vi "Find APU Channels.vi"(7 "Custom Device Ref":T1 format="%.0x", 8 "error in (no error)":errorcluster, 9 "Channel Descriptors in":T2, 11 "APU ref":T1 format="%.0x") -> (0 "error out":errorcluster, 1 "Channel Descriptors out":T2)   [LabVIEW 2011, in "Engine Sim System Explorer.lvlib"]
uses:
  Engine Sim System Explorer.lvlib
  <vilib>/NI Veristand/Custom Device API/Custom Device Item Ref.ctl
  Shared/Channel Descriptors.ctl
  Shared/FPGA Write Descriptor.ctl
  Shared/InputChannelTypes.ctl
  <vilib>/rvi/DataTransferAndStorage/Container/Common/niFpgaDataTypeControl.ctl
  Shared/FPGA Read Descriptor.ctl
  Shared/OutputChannelTypes.ctl
  Shared/Status Chan Descriptor.ctl
  <vilib>/NI Veristand/Custom Device Tools/Custom Device Utility Library/NI VeriStand - Search for Item by Name.vi
  <vilib>/NI Veristand/Custom Device Tools/Custom Device Utility Library/Custom Device Utility Library.lvlib
  Engine Simulation Shared.lvlib
  <vilib>/NI Veristand/Custom Device API/Custom Device API.lvlib
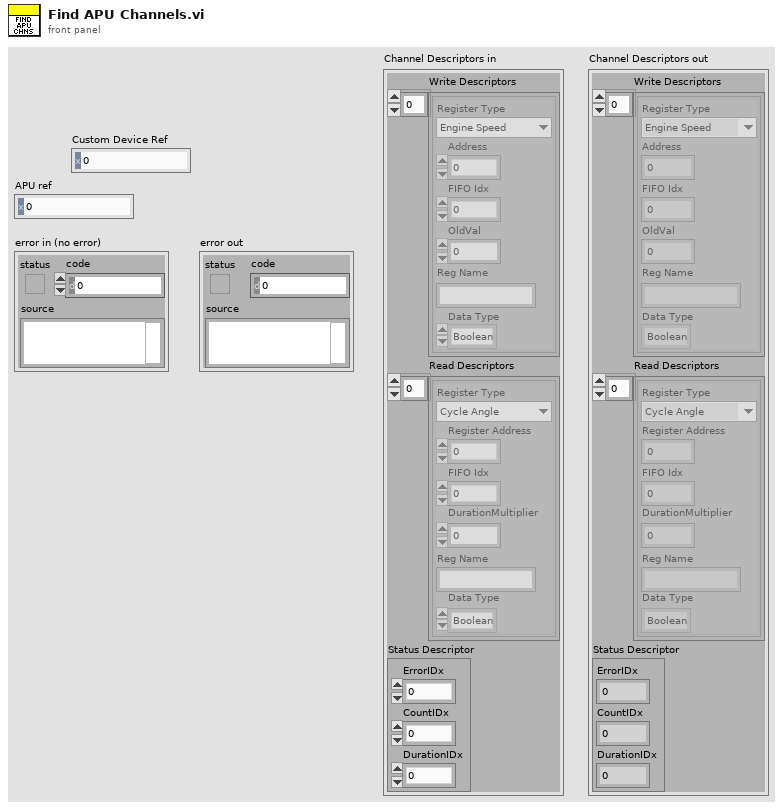
[diagram p1: front panel]
types:
  T1 = typedef "Custom Device API.lvlib/Custom Device Item Ref.ctl" = u64
  T2 = typedef "Engine Simulation Shared.lvlib/Channel Descriptors.ctl" = cluster{"Write Descriptors":T3[], "Read Descriptors":T6[], "Status Descriptor":T8}
  T3 = typedef "Engine Simulation Shared.lvlib/FPGA Write Descriptor.ctl" = cluster{"Register Type":T4, "Address":u32, "FIFO Idx":i32, "OldVal":dbl, "Reg Name":string, "Data Type":T5}
  T4 = typedef "Engine Simulation Shared.lvlib/InputChannelTypes.ctl" = enum16{"Engine Speed", "Offset"}
  T5 = typedef "niFpgaDataTypeControl.ctl" = enum32{"Boolean", "I8", "I16", "I32", "I64", "U8", "U16", "U32", "U64", "FXP", "CustomControl"}
  T6 = typedef "Engine Simulation Shared.lvlib/FPGA Read Descriptor.ctl" = cluster{"Register Type":T7, "Register Address":u32, "FIFO Idx":i32, "DurationMultiplier":dbl, "Reg Name":string, "Data Type":T5}
  T7 = typedef "Engine Simulation Shared.lvlib/OutputChannelTypes.ctl" = enum16{"Cycle Angle", "Crank Angle", "Time Duration", "Angle Duration", "Start Angle", "End Angle"}
  T8 = typedef "Engine Simulation Shared.lvlib/Status Chan Descriptor.ctl" = cluster{"ErrorIDx":i32, "CountIDx":i32, "DurationIDx":i32}
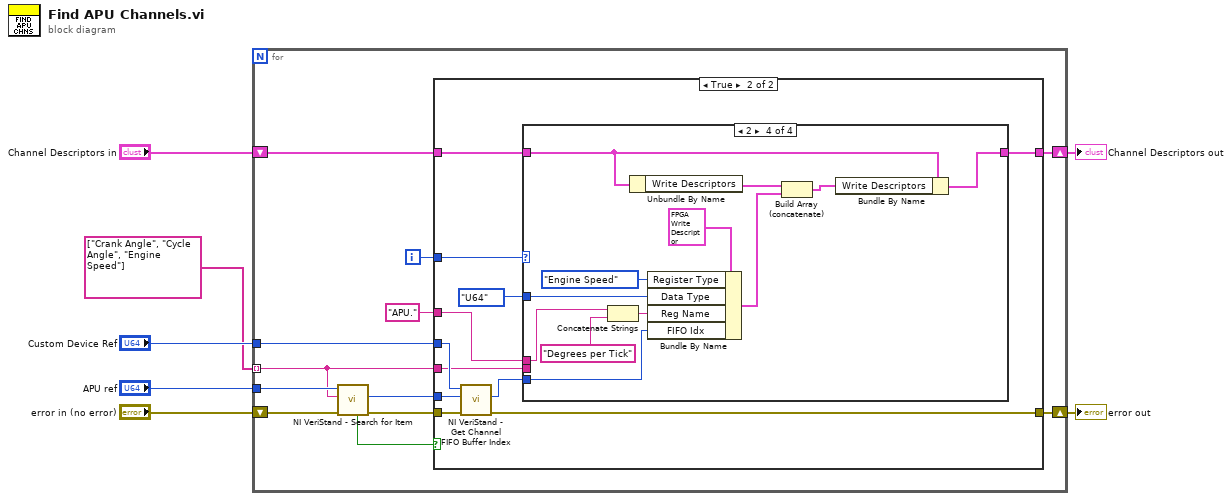
[diagram p0: block diagram]
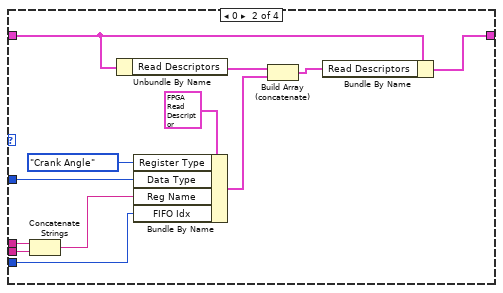
[diagram p4: hidden frame]
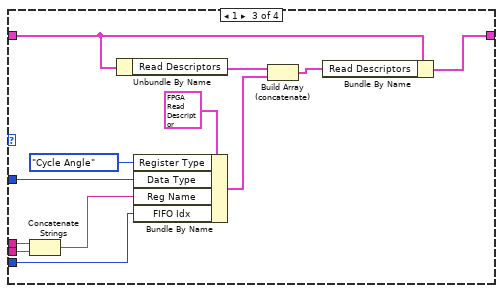
[diagram p5: hidden frame]
diagram:
  n1 = for {
    tunnel: "APU ref" -> [w19]
    tunnel: "Custom Device Ref" -> [w12]
    shift-right: [w9] -> w1
    shift-left: "error in (no error)" -> [w18]
    shift-right: [w11] -> w3
    shift-left: "Channel Descriptors in" -> [w13]
    tunnel: string[] ["Crank Angle", "Cycle Angle", "Engine Speed"] -> [w10] mode=indexing
    i -> [w8]
    n2 = call-poly <vilib>:"NI VeriStand - Search for Item.vi"("error in"=w18, "Item Name"=w10, "Section Ref in"=w19) -> ("error out"=w16:errorcluster, "Item Ref"=w15:T1, "Found"=w17:bool)  [unwired: 5 in, 1 out]
    n3 = case shown="True" w17 {
      tunnel: w16 -> [w20 w30]
      tunnel: w15 -> [_ w29]
      tunnel: "APU." ("Base path") -> [_ w22]
      tunnel: w10 -> [_ w23]
      tunnel: w13 -> [w21 w32]
      tunnel: w12 -> [_ w28]
      tunnel: [w20 w27] -> w9
      tunnel: [w21 w25] -> w11
      tunnel: w8 -> [_ w24]
      frame False {
      }
      frame True {
        n4 = call <vilib>:"NI VeriStand - Get Channel FIFO Buffer Index.vi"("error in"=w30, "Channel Ref"=w29, "Device Ref in"=w28) -> ("error out"=w27:errorcluster, "Channel FIFO Buffer Index"=w26:i32)  [unwired: 4 in, 3 out]
        n5 = case shown="2" w24 {
          tunnel: w32 -> [w33 w44 w56 w68]
          tunnel: niFpgaDataTypeControl."U64" ("Data Type") -> [_ w42 w54 w66]
          tunnel: w26 -> [_ w41 w53 w65]
          tunnel: [w33 w39 w51 w63] -> w25
          tunnel: w23 -> [_ w36 w48 _]
          tunnel: w22 -> [_ w35 w47 w61]
          frame Default {
          }
          frame 0 {
            n6 = Concatenate Strings(w35, w36) -> (w34:string)
            n7 = Unbundle By Name(w44) -> ("Read Descriptors"=w45:T6[])
            n8 = Bundle By Name(cluster=T6 {"Register Type"=enum."Cycle Angle", "Register Address"=0, "FIFO Idx"=0, "DurationMultiplier"=0.0, "Reg Name"="", "Data Type"=enum."Boolean"} ("Read Descriptor"), "Register Type"=OutputChannelTypes."Crank Angle", "Data Type"=w42, "Reg Name"=w34, "FIFO Idx"=w41) -> (w38:T6)
            n9 = Build Array (concatenate)(w45, w38) -> (w40:T6[])
            n10 = Bundle By Name(cluster=w44, "Read Descriptors"=w40) -> (w39:T2)
          }
          frame 1 {
            n11 = Concatenate Strings(w47, w48) -> (w46:string)
            n12 = Unbundle By Name(w56) -> ("Read Descriptors"=w57:T6[])
            n13 = Bundle By Name(cluster=T6 {"Register Type"=enum."Cycle Angle", "Register Address"=0, "FIFO Idx"=0, "DurationMultiplier"=0.0, "Reg Name"="", "Data Type"=enum."Boolean"} ("Read Descriptor"), "Register Type"=OutputChannelTypes."Cycle Angle", "Data Type"=w54, "Reg Name"=w46, "FIFO Idx"=w53) -> (w50:T6)
            n14 = Build Array (concatenate)(w57, w50) -> (w52:T6[])
            n15 = Bundle By Name(cluster=w56, "Read Descriptors"=w52) -> (w51:T2)
          }
          frame 2 {
            n16 = Concatenate Strings(w61, "Degrees per Tick" ("string")) -> (w60:string)
            n17 = Unbundle By Name(w68) -> ("Write Descriptors"=w69:T3[])
            n18 = Bundle By Name(cluster=T3 {"Register Type"=enum."Engine Speed", "Address"=0, "FIFO Idx"=0, "OldVal"=nan, "Reg Name"="", "Data Type"=enum."Boolean"} ("Write Descriptor"), "Register Type"=InputChannelTypes."Engine Speed", "Data Type"=w66, "Reg Name"=w60, "FIFO Idx"=w65) -> (w62:T3)
            n19 = Build Array (concatenate)(w69, w62) -> (w64:T3[])
            n20 = Bundle By Name(cluster=w68, "Write Descriptors"=w64) -> (w63:T2)
          }
        }
      }
    }
  }
  "error out" <- w1
  "Channel Descriptors out" <- w3
